vi "fix supported types and targets.vi"(8 "error in":errorcluster, 10 "DecideProjectFeatures in":refnum<class "FixedChannelTBModuleDecideFeatures.lvclass">, 11 "User Project in":refnum<vi>) -> (0 "error out":errorcluster, 3 "User Project out":refnum<vi>)   [LabVIEW 2013, in "FixedChannelTBModuleDecideFeatures.lvclass"]
uses:
  FixedChannelTBModuleDecideFeatures.lvclass
  FixedChannelTBModuleDecideFeatures.lvclass/FixedChannelTBModuleDecideFeatures.ctl
  Read supported data types.vi
  Read supported targets.vi
  Read instances allowed.vi
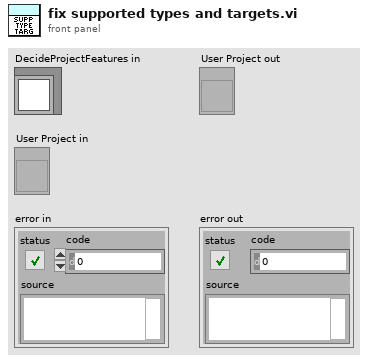
[diagram p1: front panel]
types:
  T1 = typedef "tag bus.lvlib/tag descriptor.lvclass/Data Type.ctl" = enum16{"Double", "Single", "I64", "I32", "I16", "I8", "U64", "U32", "U16", "U8", "Boolean", "String", "Array of Double", "Array of Single", "Array of I64", "Array of I32", "Array of I16", "Array of I8", "Array of U64", "Array of U32", "Array of U16", "Array of U8", "Array of Boolean", "Array of String"}
  T2 = typedef "TBM configuration.lvclass/Target Types.ctl" = enum16{"Windows", "Mac", "Linux", "Linux RT ARM", "VxWorks", "Pharlap", "Other", "Linux RT x64"}
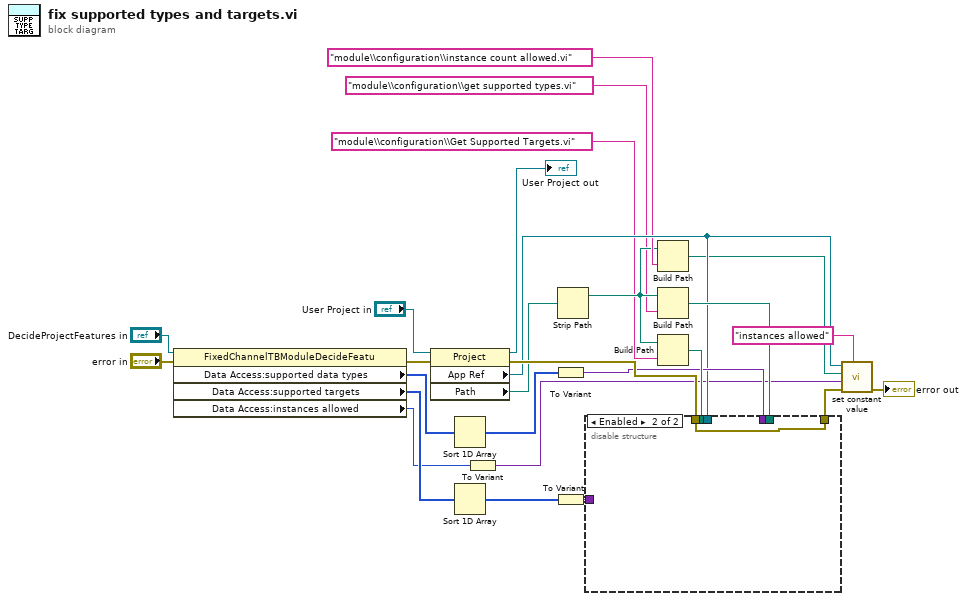
[diagram p0: block diagram]
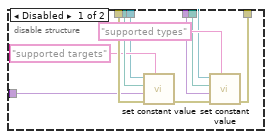
[diagram p2: hidden frame]
diagram:
  n1 = property class="FixedChannelTBModuleDecideFeatu"(reference="DecideProjectFeatures in", error in="error in") -> (error out=w20:errorcluster, "Data Access:supported data types"=w18:T1[], "Data Access:supported targets"=w19:T2[], "Data Access:instances allowed"=w9:i32)  [unwired: 1 out]
  n2 = property class="Project"(reference="User Project in", error in=w20) -> (reference out=→"User Project out":refnum<vi>, error out=w23:errorcluster, "App Ref"=w12:refnum<vi>, "Path"=w6:path)
  n3 = Sort 1D Array(array=w18) -> (sorted array=w14:T1[])
  n4 = Sort 1D Array(array=w19) -> (sorted array=w13:T2[])
  n5 = To Variant(anything=w9) -> (Variant=w8:variant)
  n6 = To Variant(anything=w14) -> (Variant=w16:variant)
  n7 = To Variant(anything=w13) -> (Variant=w17:variant)
  n8 = Strip Path(path=w6) -> (stripped path=w3:path)  [unwired: 1 out]
  n9 = Build Path(base path=w3, name or relative path="module\\configuration\\instance count allowed.vi") -> (appended path=w5:path)
  n10 = Build Path(base path=w3, name or relative path="module\\configuration\\get supported types.vi") -> (appended path=w15:path)
  n11 = Build Path(base path=w3, name or relative path="module\\configuration\\Get Supported Targets.vi") -> (appended path=w24:path)
  n12 = disable-structure shown="Enabled" {
    disable-tunnel: w24 -> [w36 _]
    disable-tunnel: w23 -> [w35 w37]
    disable-tunnel: w17 -> [w33 _]
    disable-tunnel: w16 -> [w30 _]
    disable-tunnel: w15 -> [w29 _]
    disable-tunnel: w12 -> [w28 _]
    disable-tunnel: [w27 w37] -> w11
    frame Disabled {
      n13 = call "set constant value.vi"("control name"="supported targets" ("y"), "error in"=w35, "data to set"=w33, "vi path"=w36, "Application in"=w28) -> ("error out"=w31:errorcluster)  [unwired: 6 in]
      n14 = call "set constant value.vi"("control name"="supported types" ("y"), "error in"=w31, "data to set"=w30, "vi path"=w29, "Application in"=w28) -> ("error out"=w27:errorcluster)  [unwired: 6 in]
    }
    frame Enabled {
    }
  }
  n15 = call "set constant value.vi"("control name"="instances allowed", "error in"=w11, "data to set"=w8, "vi path"=w5, "Application in"=w12) -> ("error out"=→"error out":errorcluster)  [unwired: 6 in]
